vi "Initialize Logging.vi"(7 "Timestamp":bool, 8 "error in":errorcluster, 9 "log thresholds":T1 {"Segment Files By" items=["Time", "Size"]}, 10 "Base name":string, 11 "Log File Directory":string) -> (0 "error out":errorcluster, 2 "File path out":path, 3 "Log Producer out":T2)   [LabVIEW 2020, in "AIM ARINC 664 Engine.lvlib" / "Implementation.lvlib" / "Monitor Execution Unit.lvclass"]
uses:
  Monitor Execution Unit.lvclass
  Monitor Execution Unit.lvclass/Monitor Execution Unit.ctl
  Logging/Frame Logging/Frame Logging.lvlib
  Logging/Frame Logging/Log_Producer.ctl
  Logging/Frame Logging/Message_Request_Action.ctl
  Logging/Frame Logging/Message_Request.ctl
  Shared/loggingThreshold_types.ctl
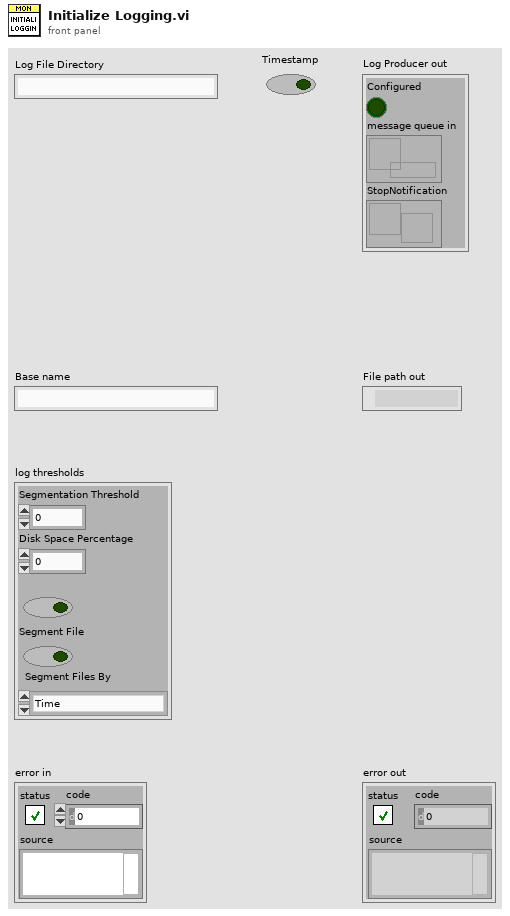
[diagram p1: front panel]
types:
  T1 = typedef "loggingThreshold_types.ctl" = cluster{"Segmentation Threshold":dbl, "Disk Space Percentage":dbl, "Check Disk Space":bool, "Segment File":bool, "Segment Files By":u16}
  T2 = typedef "Frame Logging.lvlib/Log_Producer.ctl" = cluster{"Configured":bool, "message queue in":refnum<queue>, "StopNotification":refnum<notifier>}
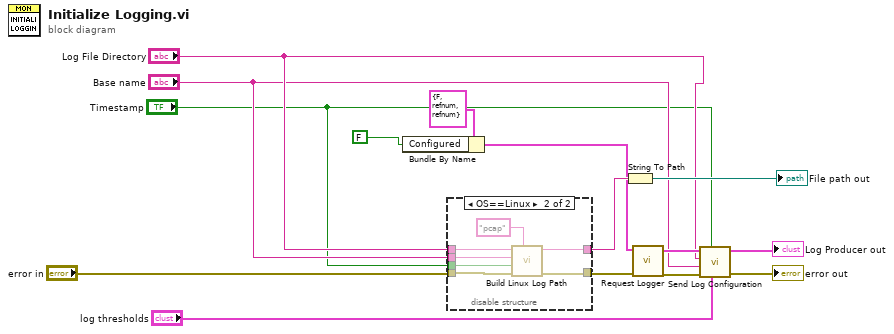
[diagram p0: block diagram]
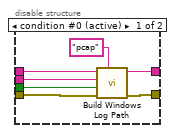
[diagram p2: hidden frame]
diagram:
  n1 = Bundle By Name(cluster=T2 {"Configured"=FALSE, "message queue in"=refnum, "StopNotification"=refnum} ("Log Producer out"), "Configured"=FALSE) -> (w10:T2)
  n2 = disable-structure shown="OS==Linux" {
    disable-tunnel: [w20 w23] -> w15
    disable-tunnel: [w19 w24] -> w13
    disable-tunnel: "error in" -> [w18 w25]
    disable-tunnel: "Log File Directory" -> [w21 w28]
    disable-tunnel: "Base name" -> [w16 w27]
    disable-tunnel: "Timestamp" -> [w17 w26]
    frame condition #0 (active) {
      n3 = call "Build Windows Log Path.vi"("Extension"="pcap", "error in (no error)"=w18, "Timestamp"=w17, "Name"=w16, "Log File Directory"=w21) -> ("error out"=w19:errorcluster, "Log File Path"=w20:string)  [unwired: 5 in]
    }
    frame condition #1 {
      n4 = call "Build Linux Log Path.vi"("Extension"="pcap", "error in (no error)"=w25, "Timestamp"=w26, "Name"=w27, "Log File Directory"=w28) -> ("error out"=w24:errorcluster, "Log File Path"=w23:string)  [unwired: 5 in]
    }
  }
  n5 = String To Path(string=w15) -> (path=→"File path out":path)
  n6 = call "Request Logger.vi"("error in (no error)"=w13, "Log Producer in"=w10) -> ("error out"=w1:errorcluster, "Log Producer out"=w8:T2)  [unwired: 8 in]
  n7 = call "Send Log Configuration.vi"("log thresholds"="log thresholds", "Timestamp"="Timestamp", "error in"=w1, "Base name"="Base name", "Log File Directory"="Log File Directory", "Log Producer in"=w8) -> ("error out"=→"error out":errorcluster, "Log Producer out"=→"Log Producer out":T2)  [unwired: 4 in]
